vi "Build Element Tree.vi"(7 "Hierarchies":cluster{"Hierarchy":string[]}[](array[cluster]), 8 "error in (no error)":errorcluster, 10 "Elements in":T1[](array[typedef]), 11 "Config Manager in":refnum<class "Config Manager.lvclass">) -> (0 "error out":errorcluster, 3 "Config Manager out":refnum<class "Config Manager.lvclass">)   [LabVIEW 2023, in "CDM-Config.lvlib" / "Config Manager.lvclass"]
uses:
  Config Manager.lvclass
  Config Element/Element Data.ctl
  Node Info.ctl
  Meta Data.ctl
  Value Type.ctl
  Config Element/Config Element.lvclass
  Config Manager.lvclass/Config Manager.ctl
  Create Missing Element.vi
  Build Hierarchy Map.vi
  CDM-Config.lvlib
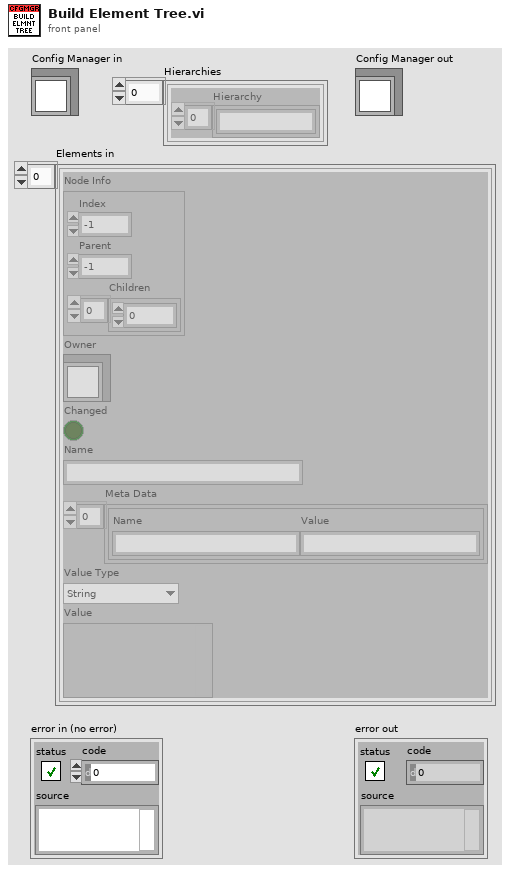
[diagram p1: front panel]
types:
  T1 = typedef "CDM-Config.lvlib/Config Element.lvclass/Element Data.ctl" = cluster{"Node Info":T2, "Owner":refnum<class>, "Changed":bool, "Name":string, "Meta Data":T3[], "Value Type":T4, "Value":variant}
  T2 = typedef "CDM-Config.lvlib/Node Info.ctl" = cluster{"Index":i32, "Parent":i32, "Children":i32[]}
  T3 = typedef "CDM-Config.lvlib/Meta Data.ctl" = cluster{"Name":string, "Value":string}
  T4 = typedef "CDM-Config.lvlib/Value Type.ctl" = enum16{"String", "Number", "Bool", "Object", "Array"}
  T5 = typedef "CDM-Config.lvlib/Config Manager.lvclass/Ref Data.ctl" = cluster{"Elements":refnum<class "Config Element.lvclass">[], "Hierarchy Map":map{string[], i32}, "Element Map":map{refnum<class "Config Element.lvclass">, i32}}
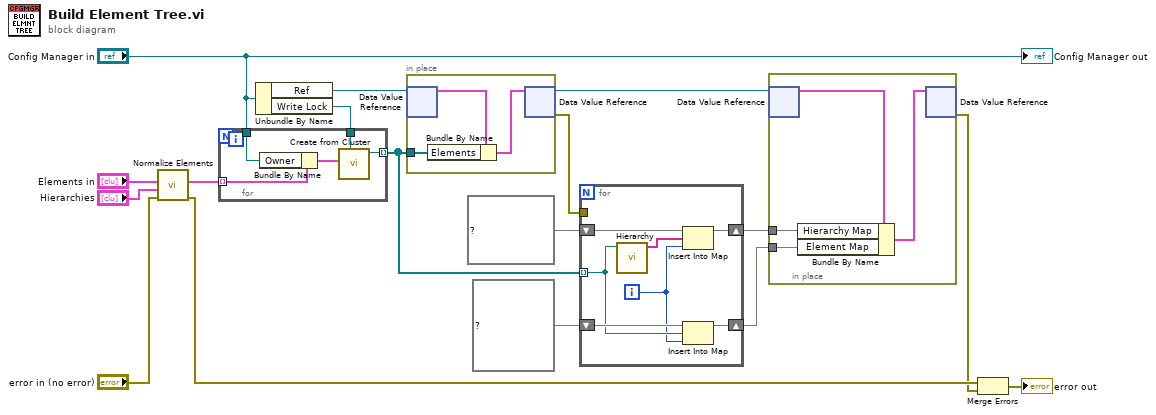
[diagram p0: block diagram]
diagram:
  n1 = call "Normalize Elements.vi"("error in (no error)"="error in (no error)", "Hierarchies"="Hierarchies", "Elements in"="Elements in") -> ("error out"=w15:errorcluster, "Elements"=w12:T1[])  [unwired: 7 in]
  n2 = Unbundle By Name("Config Manager in") -> ("Ref"=w5:refnum<data-value>, "Write Lock"=w1:refnum<notifier>)
  n3 = for {
    tunnel: w12 -> [w22] mode=indexing
    tunnel: "Config Manager in" -> [w21]
    tunnel: [w19] -> w2 mode=indexing
    tunnel: w1 -> [w18]
    n4 = Bundle By Name(cluster=w22, "Owner"=w21) -> (w20:T1)
    n5 = call "Create from Cluster.vi"("Write Lock"=w18, "Ref Data"=w20) -> ("Config Element out"=w19:refnum<class "Config Element.lvclass">)  [unwired: 8 in, 1 out]
  }
  n6 = in-place {
    in-place-border: w2 -> [w23]
    n7 = in-place-dvr #1(w5) -> (w25:T5)  [unwired: 1 out]
    n8 = Bundle By Name(cluster=w25, "Elements"=w23) -> (w24:T5)
    n9 = in-place-dvr #1(w24) -> (w4:refnum<data-value>, w3:errorcluster)
  }
  n10 = for {
    tunnel: w2 -> [w28] mode=indexing
    shift-right: [w30] -> w13
    shift-left: map{string[], i32} {} ("Hierarchy Map") -> [w32]
    shift-right: [w27] -> w7
    shift-left: map{refnum<class "Config Element.lvclass">, i32} {} ("Hierarchy Map") -> [w29]
    tunnel: w3 -> [_]
    i -> [w26]
    n11 = call "Hierarchy.vi"("Config Element in"=w28) -> ("Hierarchy"=w31:string[])  [unwired: 9 in, 1 out]
    n12 = Insert Into Map(map in=w32, key=w31, value=w26) -> (map out=w30:map{string[], i32})  [unwired: 2 out]
    n13 = Insert Into Map(map in=w29, key=w28, value=w26) -> (map out=w27:map{refnum<class "Config Element.lvclass">, i32})  [unwired: 2 out]
  }
  n14 = in-place {
    in-place-border: w13 -> [w34]
    in-place-border: w7 -> [w33]
    n15 = in-place-dvr #2(w4) -> (w36:T5)  [unwired: 1 out]
    n16 = Bundle By Name(cluster=w36, "Hierarchy Map"=w34, "Element Map"=w33) -> (w35:T5)
    n17 = in-place-dvr #2(w35) -> (w8:errorcluster)  [unwired: 1 out]
  }
  n18 = Merge Errors(w15, w8) -> (→"error out":errorcluster)
  "Config Manager out" <- "Config Manager in"
